vi "TimingSource UI.vi"() -> ()   [LabVIEW 2019, in "TimingSource.lvclass"]
uses:
  TimingSource.lvclass
  <vilib>/NI/Configuration Framework/Node/NodeRef.ctl
  <vilib>/NI/Configuration Framework/Node/NISE_CEF_Node.lvclass
  <vilib>/NI/AMC/Message Queue.ctl
  <vilib>/NI/AMC/Message.ctl
  <vilib>/NI/Tools/Keyed Array/KeyedArray.ctl
  <vilib>/NI/Configuration Framework/Node/UserEventRef.ctl
  <vilib>/NI/Configuration Framework/Controls/EventCluster.ctl
  C:/Program Files (x86)/National Instruments/LabVIEW 2019/vi.lib/NI/Configuration Framework/Node/NISE_CEF_Node.lvclass
  TimingSource.lvclass/TimingSource.ctl
  Read Timing Source Properties.vi
  Write Timing Source Properties.vi
  <vilib>/NI/AMC/Create Single Message.vi
  <vilib>/NI/AMC/Update Message Routing Info.vi
  <vilib>/NI/AMC/Send Message.vi
  <vilib>/NI/AMC/AMC.lvlib
  Configuration Tool.lvlib
  <vilib>/NI/Tools/Keyed Array/Tools_KeyedArray.lvlib
  <vilib>/NI/Configuration Framework/NISE_CEF_TreeControl.lvlib
panel:
  in  "Main UI Tab":enum32{"Timing Source"}(tab)
  in  "Supported Targets":i32(listbox)
  in  "Host Path to selected Target's Timing Source VI":path
  in  "Real Time System Destination":string
  in  "user event":T1
  in  "main queue":T2
  in  "node ref":T3
  # "Target Information"
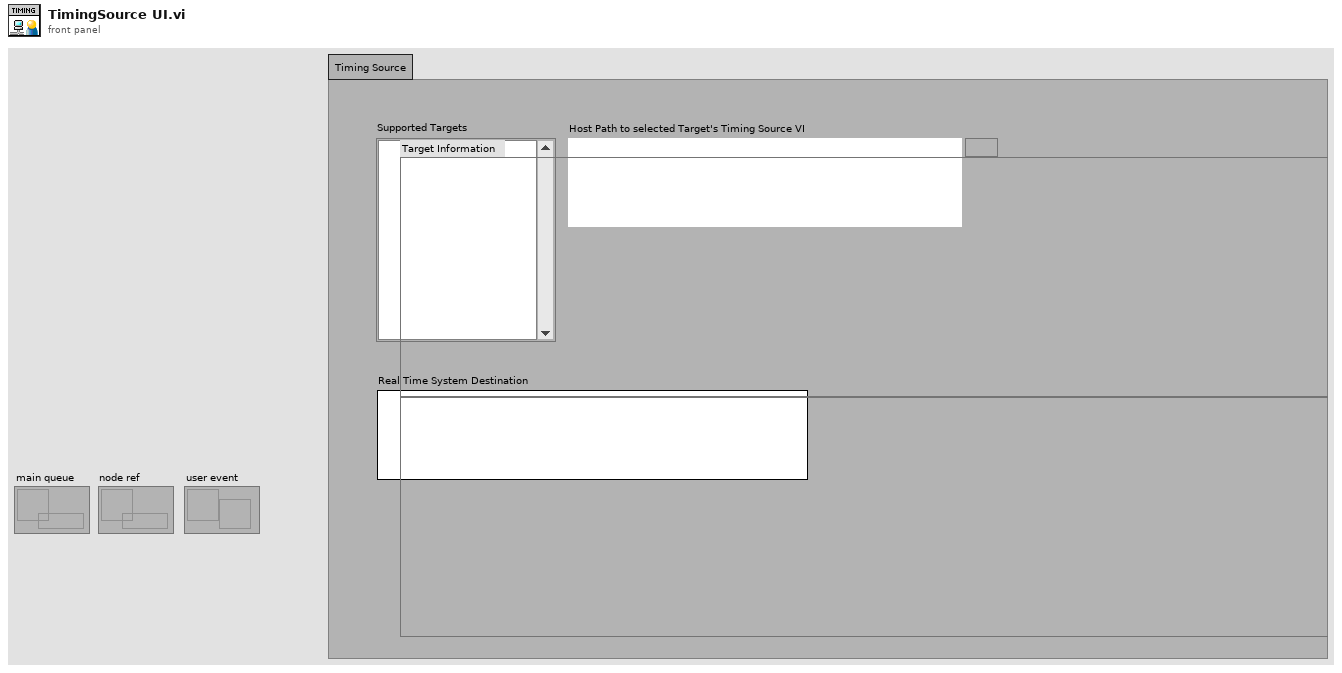
[diagram p1: front panel]
types:
  T1 = typedef "NISE_CEF_Node.lvclass/UserEventRef.ctl" = refnum<user-event>
  T2 = typedef "AMC.lvlib/Message Queue.ctl" = refnum<queue>
  T3 = typedef "NISE_CEF_Node.lvclass/NodeRef.ctl" = refnum<data-value>
  T4 = typedef "Timing Source Properties.ctl" = cluster{"Has Timing Source Capability":bool, "Source Distribution":T5}
  T5 = typedef "Source Distribution for TimingSource.ctl" = cluster{"Supported Target":T6, "Source":T7, "Real Time System Destination":string, "Version":string}[]
  T6 = typedef "Target.ctl" = enum16{"All", "Pharlap", "VxWorks", "Windows", "Linux_32_ARM", "Linux_x64", "PharlapWindows", "PharlapVxWorks", "VxWorksWindows"}
  T7 = typedef "Path Cluster.ctl" = cluster{"Path":path, "Path Type":enum16{"Absolute", "To Base", "To Common Doc Dir", "To Application Data Dir"}}
  T8 = enum16{"Absolute", "To Base", "To Common Doc Dir", "To Application Data Dir"}
  T9 = cluster{"appended path":path, "Real Time System Destination":string}
  T10 = cluster{"Supported Target":T6, "Source":T7, "Real Time System Destination":string, "Version":string}
  T11 = cluster{"appended path":path, "Real Time System Destination":string}[]
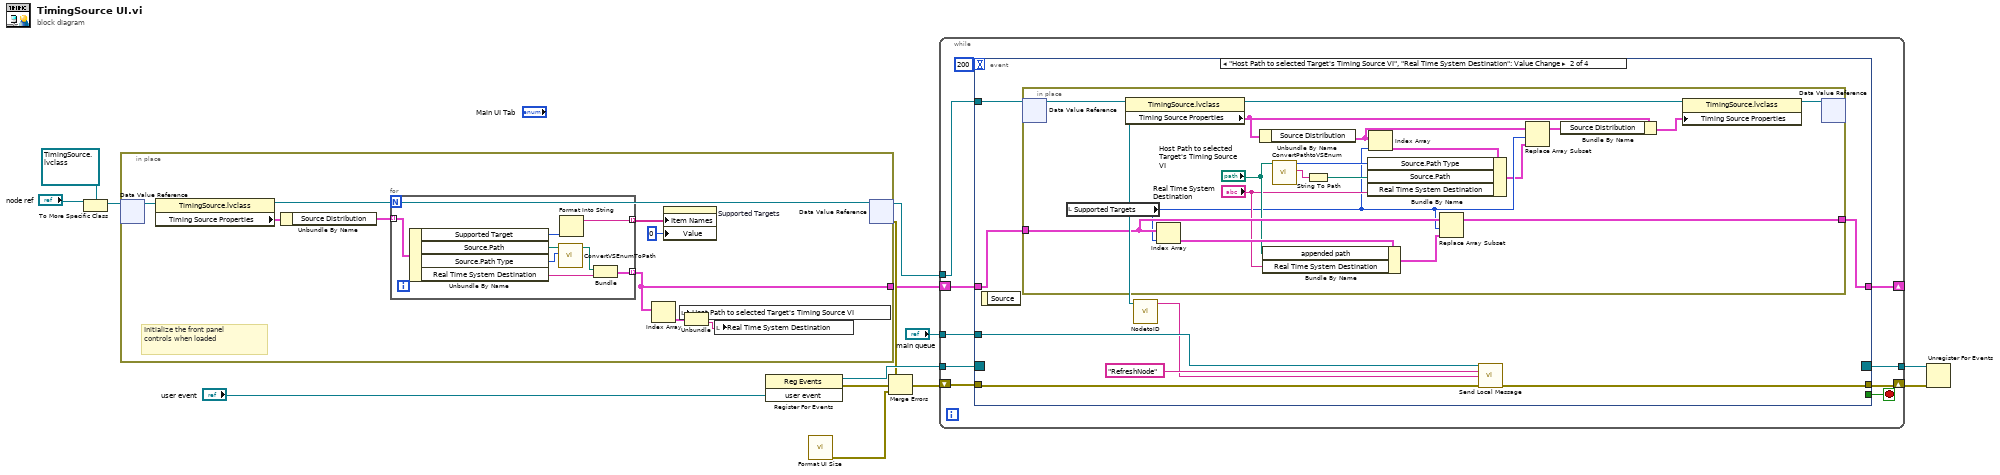
[diagram p0: block diagram]
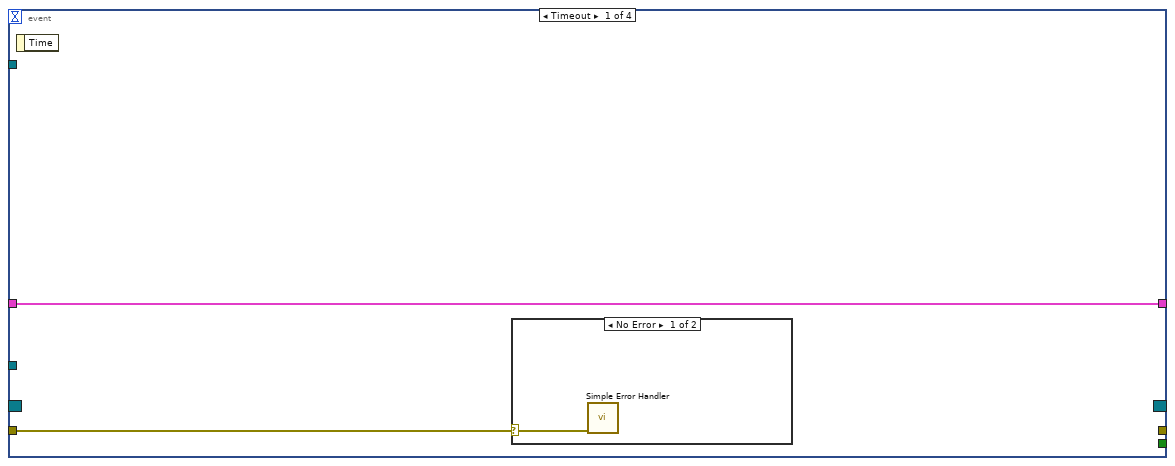
[diagram p2: hidden frame]
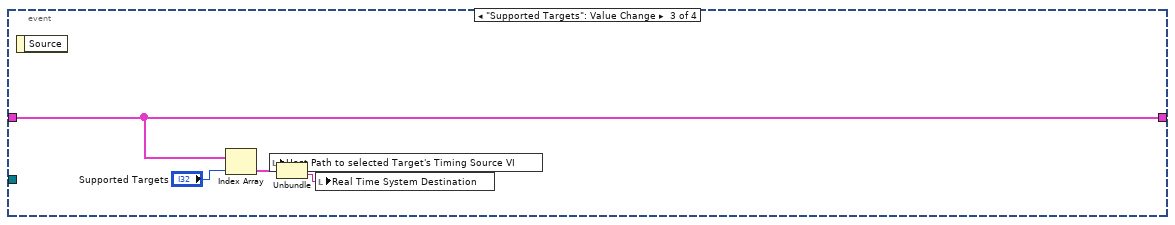
[diagram p4: hidden frame]
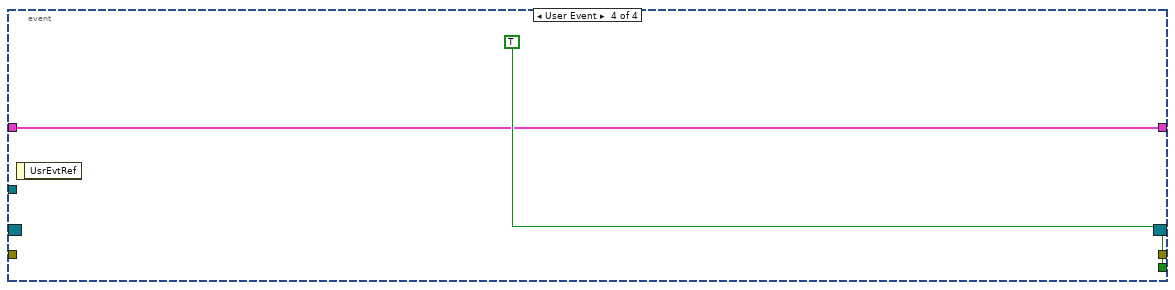
[diagram p5: hidden frame]
diagram:
  n1 = To More Specific Class(target class=refnum<data-value> refnum ("data value reference"), reference="node ref") -> (specific class reference=w7:refnum<data-value>)  [unwired: 1 in, 1 out]
  n2 = in-place {
    in-place-border: [w15] -> w2
    # "Initialize the front panel controls when loaded"
    n3 = in-place-dvr #1(w7) -> (w24:refnum<class "TimingSource.lvclass">)  [unwired: 1 out]
    n4 = property class="TimingSource.lvclass"(reference=w24) -> (reference out=w23:refnum<class "TimingSource.lvclass">, "Timing Source Properties"=w22:T4)  [unwired: 1 in, 1 out]
    n5 = Unbundle By Name(w22) -> ("Source Distribution"=w21:T5)
    n6 = for {
      tunnel: w21 -> [w32] mode=indexing
      tunnel: [w30] -> w20 mode=indexing
      tunnel: [w25] -> w15 mode=indexing
      n7 = Unbundle By Name(w32) -> ("Supported Target"=w31:T6, "Source.Path"=w29:path, "Source.Path Type"=w28:T8, "Real Time System Destination"=w26:string)
      n8 = call "ConvertVSEnumToPath.vi"("Source.Path Type"=w28, "Path In"=w29) -> ("appended path"=w27:path)  [unwired: 9 in]
      n9 = Format Into String(w31) -> (resulting string=w30:string)  [unwired: 3 in, 1 out]
      n10 = Bundle("appended path"=w27, "Real Time System Destination"=w26) -> (w25:T9)  [unwired: 1 in]
    }
    n11 = Index Array(array=w15) -> (element=w18:T9)  [unwired: 1 in]
    n12 = property on="Supported Targets" class="LstBox (strict)"("Item Names"=w20, "Value"=0 ("Selection Mode")) -> ()  [unwired: 2 in, 2 out]
    n13 = Unbundle(w18) -> ("appended path"=w17:path, "Real Time System Destination"=w16:string)
    n14 = local write "Host Path to selected Target's Timing Source VI"(w17) -> ()
    n15 = local write "Real Time System Destination"(w16) -> ()
    n16 = in-place-dvr #1(w23) -> (w14:refnum<data-value>, w4:errorcluster)
  }
  n17 = register-events("user event") -> (reference out=w11:refnum<event-registration>, error out=w5:errorcluster)  [unwired: 2 in]
  n18 = call "Format UI Size.vi"() -> ("error out"=w1:errorcluster)  [unwired: 11 in]
  n19 = Merge Errors(w4, w5, w1) -> (w3:errorcluster)
  n20 = while {
    tunnel: w14 -> [w42]
    tunnel: "main queue" -> [w41]
    tunnel: w11 -> [w39]
    tunnel: [w38] -> w10
    shift-right: [w36] -> w9
    shift-left: w3 -> [w35]
    shift-right: [w33] -> _
    shift-left: w2 -> [w34]
    stop <- w37 stop-if-true
    n21 = event shown="[1] \"Host Path to selected Target's Timing Source VI\", \"Real Time System Destination\": Value Change" {
      selector: w39 -> [_ _ _ _]
      dyn-events: [_ _ _ _] -> w38
      timeout: 200 -> [_ _ _ _]
      tunnel: w42 -> [_ w51 _ _]
      tunnel: w41 -> [_ w52 _ _]
      tunnel: [_ _ _ TRUE] -> w37
      tunnel: [_ w49 _ _] -> w36
      tunnel: w35 -> [w44 w48 _ _]
      tunnel: w34 -> [w43 w47 w73 w78]
      tunnel: [w43 w46 w73 w78] -> w33
      event Timeout {
        n22 = event-data() -> ()  [unwired: 1 in, 1 out]
        n23 = case shown="No Error" w44 {
          selector: w44 -> [w45 _]
          frame No Error {
            n24 = call <vilib>:"Simple Error Handler.vi"("error in (no error)"=w45) -> ()  [unwired: 4 in, 5 out]
          }
          frame Error {
          }
        }
      }
      event "Host Path to selected Target's Timing Source VI", "Real Time System Destination": Value Change {
        n25 = event-data() -> ()  [unwired: 1 in, 1 out]
        n26 = in-place {
          in-place-border: w47 -> [w70]
          in-place-border: [w68] -> w46
          n27 = in-place-dvr #2(w51) -> (w72:refnum<class "TimingSource.lvclass">)  [unwired: 1 out]
          n28 = local read "Supported Targets"() -> (w60:i32)
          n29 = property class="TimingSource.lvclass"(reference=w72) -> (reference out=w56:refnum<class "TimingSource.lvclass">, "Timing Source Properties"=w58:T4)  [unwired: 1 in, 1 out]
          n30 = Index Array(array=w70, index=w60) -> (element=w71:T9)
          n31 = Unbundle By Name(w58) -> ("Source Distribution"=w61:T5)
          n32 = Bundle By Name(cluster=w71, "appended path"="Host Path to selected Target's Timing Source VI", "Real Time System Destination"="Real Time System Destination") -> (w69:T9)
          n33 = call "ConvertPathtoVSEnum.vi"("Path In"="Host Path to selected Target's Timing Source VI") -> ("Remaining Path"=w64:string, "VS Enum Out"=w65:T8)  [unwired: 9 in]
          n34 = String To Path(string=w64) -> (path=w63:path)
          n35 = Index Array(array=w61, index=w60) -> (element=w67:T10)
          n36 = Bundle By Name(cluster=w67, "Source.Path Type"=w65, "Source.Path"=w63, "Real Time System Destination"="Real Time System Destination") -> (w59:T10)
          n37 = Replace Array Subset(array=w70, new element=w69, index=w60) -> (w68:T11)
          n38 = Replace Array Subset(array=w61, new element=w59, index=w60) -> (w57:T5)
          n39 = Bundle By Name(cluster=w58, "Source Distribution"=w57) -> (w55:T4)
          n40 = property class="TimingSource.lvclass"(reference=w56, "Timing Source Properties"=w55) -> (reference out=w54:refnum<class "TimingSource.lvclass">)  [unwired: 1 in, 1 out]
          n41 = in-place-dvr #2(w54) -> ()  [unwired: 2 out]
        }
        n42 = call <vilib>:"NodetoID.vi"("node ref"=w51) -> ("ID"=w50:string)  [unwired: 9 in, 1 out]
        n43 = call <vilib>:"Send Local Message.vi"("message queue in"=w52, "message name"="RefreshNode" ("Message Name"), "message value"=w50, "error in"=w48) -> ("error out"=w49:errorcluster)  [unwired: 9 in, 2 out]
      }
      event "Supported Targets": Value Change {
        n44 = event-data() -> ()  [unwired: 1 in, 1 out]
        n45 = Index Array(array=w73, index="Supported Targets") -> (element=w74:T9)
        n46 = Unbundle(w74) -> ("appended path"=w75:path, "Real Time System Destination"=w76:string)
        n47 = local write "Host Path to selected Target's Timing Source VI"(w75) -> ()
        n48 = local write "Real Time System Destination"(w76) -> ()
      }
      event User Event {
        n49 = event-data() -> ()  [unwired: 1 in, 1 out]
      }
    }
  }
  n50 = Unregister For Events(event registration refnum=w10, error in=w9) -> ()  [unwired: 1 out]
